vi "svx_Oct_Transparency Write.vi"(4 "error in (no error)":errorcluster, 5 "Value":bool, 6 "Container State":T2, 7 "Display State In":T1={"X Scale Width %"=50.0, "Y Scale Height %"=50.0, "X-Axis Range"={"Minimum"=0.0, "Maximum"=10.0}, "Y-Axis Range"={"Minimum"=0.0, "Maximum"=10.0}, "Z-Axis Range"={"Minimum"=0.0, "Maximum"=10.0}, "Plot Color"=0, "Frame Color"=61212, "Background Color"=16252785, "Initial AutoScale Y"=TRUE, "AutoScale X"=2, "AutoScale Y"=2, "AutoScale Z"=2, "Plot Transparency"=FALSE, "X-Axis Name"="Frequency", "Y-Axis Name"="Amplitude", "Z-Axis Name"="", "X-Axis Scaling Factor"={"Offset"=0.0, "Multiplier"=1.0}, "Y-Axis Scaling Factor"={"Offset"=0.0, "Multiplier"=1.0}, "Z-Axis Scaling Factor"={"Offset"=0.0, "Multiplier"=1.0}, "X-Scale Visible"=TRUE, "Y-Scale Visible"=TRUE, "Z-Scale Visible"=TRUE, "X-Scale Label Visible"=TRUE, "Y-Scale Label Visible"=TRUE, "Z-Scale Label Visible"=TRUE, "X-Axis Range Scaled"={"Minimum"=0.0, "Maximum"=10.0}, "Y-Axis Range Scaled"={"Minimum"=0.0, "Maximum"=10.0}, "Z-Axis Range Scaled"={"Minimum"=0.0, "Maximum"=10.0}, "Rev Z Order"=FALSE, "X-Scale Format Str"="%#.4g", "Y-Scale Format Str"="%#.4g", "Z-Scale Format Str"="%#.4g", "Decor color"=12369084, "Scale Range Change"=refnum, "out of state queue"=refnum, "property nodes"=refnum}) -> (0 "error out":errorcluster, 3 "Display State Out":T1={"X Scale Width %"=50.0, "Y Scale Height %"=50.0, "X-Axis Range"={"Minimum"=0.0, "Maximum"=10.0}, "Y-Axis Range"={"Minimum"=0.0, "Maximum"=10.0}, "Z-Axis Range"={"Minimum"=0.0, "Maximum"=10.0}, "Plot Color"=0, "Frame Color"=61212, "Background Color"=16252785, "Initial AutoScale Y"=TRUE, "AutoScale X"=2, "AutoScale Y"=2, "AutoScale Z"=2, "Plot Transparency"=FALSE, "X-Axis Name"="Frequency", "Y-Axis Name"="Amplitude", "Z-Axis Name"="", "X-Axis Scaling Factor"={"Offset"=0.0, "Multiplier"=1.0}, "Y-Axis Scaling Factor"={"Offset"=0.0, "Multiplier"=1.0}, "Z-Axis Scaling Factor"={"Offset"=0.0, "Multiplier"=1.0}, "X-Scale Visible"=TRUE, "Y-Scale Visible"=TRUE, "Z-Scale Visible"=TRUE, "X-Scale Label Visible"=TRUE, "Y-Scale Label Visible"=TRUE, "Z-Scale Label Visible"=TRUE, "X-Axis Range Scaled"={"Minimum"=0.0, "Maximum"=10.0}, "Y-Axis Range Scaled"={"Minimum"=0.0, "Maximum"=10.0}, "Z-Axis Range Scaled"={"Minimum"=0.0, "Maximum"=10.0}, "Rev Z Order"=FALSE, "X-Scale Format Str"="%#.4g", "Y-Scale Format Str"="%#.4g", "Z-Scale Format Str"="%#.4g", "Decor color"=12369084, "Scale Range Change"=refnum, "out of state queue"=refnum, "property nodes"=refnum})   [LabVIEW 2017, in "SVX Octave Waterfall Graph.xctl"]
uses:
  <vilib>/addons/_XControls/Octave Waterfall Graph/SVX Octave Waterfall Graph.xctl
  <vilib>/_xctls/Container State.ctl
  <vilib>/addons/_XControls/Octave Waterfall Graph/subVIs/svx_Oct_Waterfall State.ctl
  <vilib>/_xctls/XControlSupport.lvlib
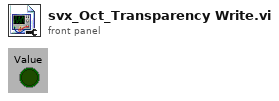
[diagram p1: front panel]
types:
  T1 = typedef "SVX Octave Waterfall Graph.xctl/svx_Oct_Waterfall State.ctl" = cluster{"X Scale Width %":dbl, "Y Scale Height %":dbl, "X-Axis Range":cluster{"Minimum":dbl, "Maximum":dbl}, "Y-Axis Range":cluster{"Minimum":dbl, "Maximum":dbl}, "Z-Axis Range":cluster{"Minimum":dbl, "Maximum":dbl}, "Plot Color":u32, "Frame Color":u32, "Background Color":u32, "Initial AutoScale Y":bool, "AutoScale X":u8, "AutoScale Y":u8, "AutoScale Z":u8, "Plot Transparency":bool, "X-Axis Name":string, "Y-Axis Name":string, "Z-Axis Name":string, "X-Axis Scaling Factor":cluster{"Offset":dbl, "Multiplier":dbl}, "Y-Axis Scaling Factor":cluster{"Offset":dbl, "Multiplier":dbl}, "Z-Axis Scaling Factor":cluster{"Offset":dbl, "Multiplier":dbl}, "X-Scale Visible":bool, "Y-Scale Visible":bool, "Z-Scale Visible":bool, "X-Scale Label Visible":bool, "Y-Scale Label Visible":bool, "Z-Scale Label Visible":bool, "X-Axis Range Scaled":cluster{"Minimum":dbl, "Maximum":dbl}, "Y-Axis Range Scaled":cluster{"Minimum":dbl, "Maximum":dbl}, "Z-Axis Range Scaled":cluster{"Minimum":dbl, "Maximum":dbl}, "Rev Z Order":bool, "X-Scale Format Str":string, "Y-Scale Format Str":string, "Z-Scale Format Str":string, "Decor color":u32, "Scale Range Change":refnum<user-event>, "out of state queue":refnum<queue>, "property nodes":refnum<queue>}
  T2 = typedef "XControlSupport.lvlib/Container State.ctl" = cluster{"Indicator?":bool, "Run Mode?":bool, " Refnum":refnum<vi>}
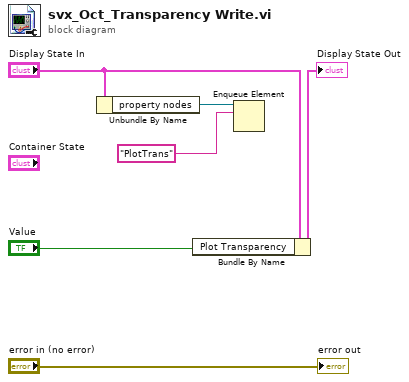
[diagram p0: block diagram]
diagram:
  n1 = Unbundle By Name("Display State In") -> ("property nodes"=w3:refnum<queue>)
  n2 = Bundle By Name(cluster="Display State In", "Plot Transparency"="Value") -> (→"Display State Out":T1)
  n3 = Enqueue Element(queue=w3, element="PlotTrans" ("Property Name")) -> ()  [unwired: 2 in, 3 out]
  "error out" <- "error in (no error)"
